vi "insert standard into cycle.vi"(1 "error out 2":errorcluster) -> (0 "error out":errorcluster)   [LabVIEW 2016]
panel:
  out "Array 2":dbl[][](array[numeric])
  out "Array":dbl[](array[numeric])
  out "sequence  Result":dbl[][](array[numeric])
  out "cycle results dbl":dbl[][](array[numeric])
  out "cycle results labels":string[](array[string])
  out "Cycle data by position":dbl[][][](array[numeric])
  out "Final Result":string[][](array[string])
  out "cycle result header":string[](array[string])
  out "sequence result header":string[](array[string])
  out "Final result header":string[](array[string])
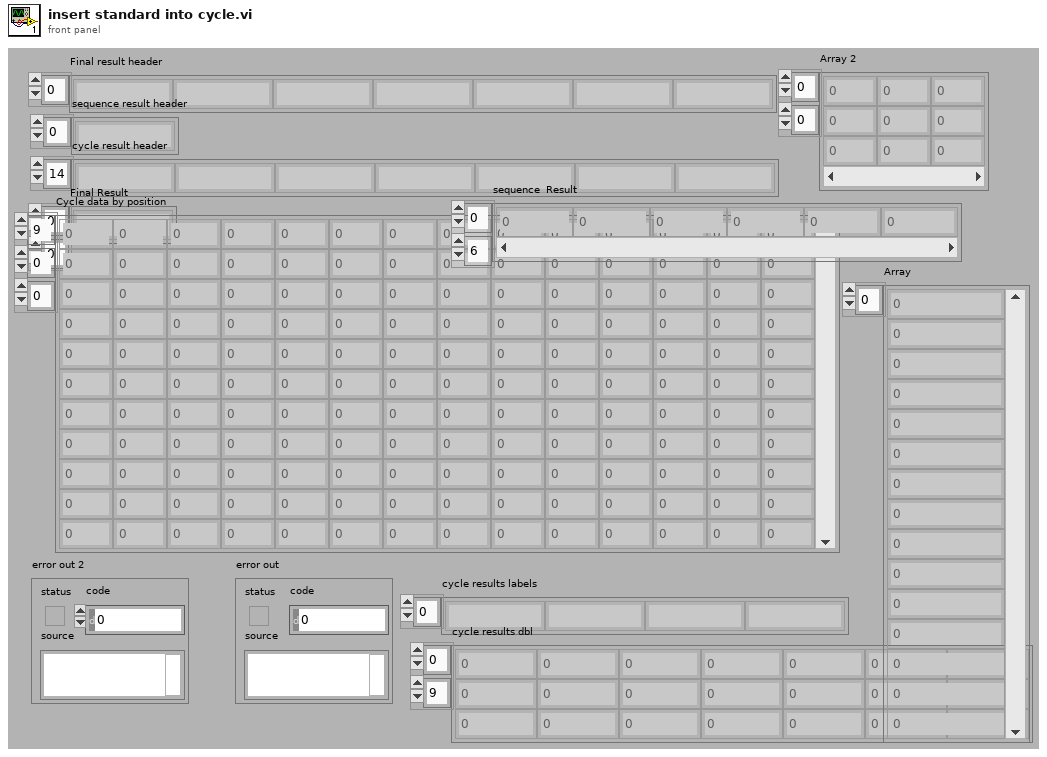
[diagram p1: front panel]
types:
  T1 = typedef "cycle results control.ctl" = cluster{"sample info":string[][], "cycle results labels":string[], "cycle results dbl":dbl[][]}
  T2 = typedef "data control cluster.ctl" = cluster{"Final result header":string[], "sequence result header":string[], "cycle result header ":string[], "Final Result":string[][], "sequence  Result":dbl[][], "Cycle data by seq":dbl[][][], "Cycle data by position":dbl[][][], "Final seq  Result":dbl[][], "only specific type":dbl[][]}
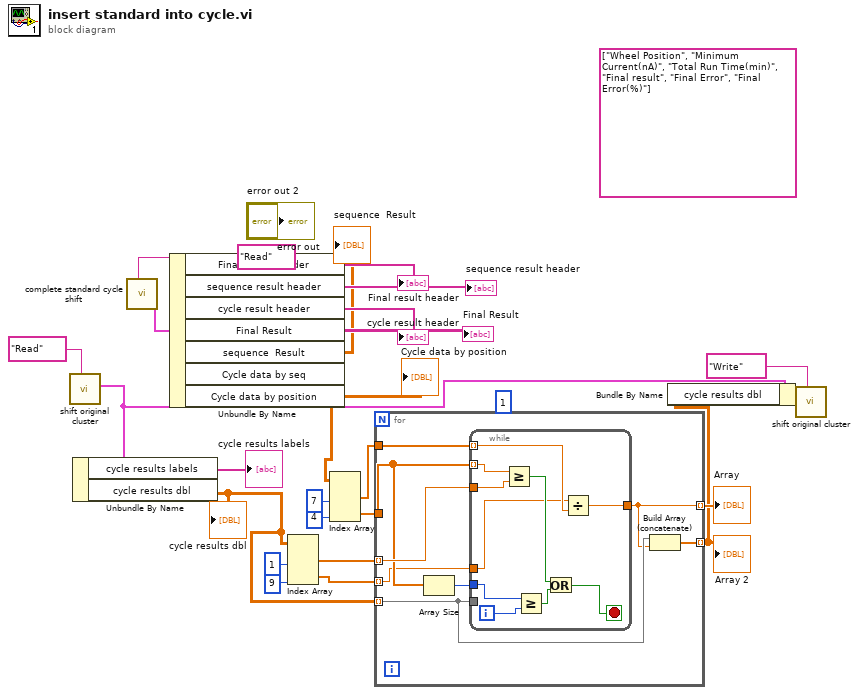
[diagram p0: block diagram]
diagram:
  (unwired) string[] ["Wheel Position", "Minimum Current(nA)", "Total Run Time(min)", "Final result", "Final Error", "Final Error(%)"]
  (unwired) 1 ("disabled index (col)")
  n1 = call "shift original cluster.vi"("read write shift"="Read") -> ("cycle results cluster out"=w3:T1)  [unwired: 9 in, 1 out]
  n2 = Unbundle By Name(w3) -> ("cycle results labels"=→"cycle results labels":string[], "cycle results dbl"=w10:dbl[][])
  "cycle results dbl" <- w10
  n3 = call "complete standard cycle shift.vi"("read write shift"="Read") -> ("DATA CLUSTER out"=w23:T2)  [unwired: 9 in, 1 out]
  n4 = Unbundle By Name(w23) -> ("Final result header"=→"Final result header":string[], "sequence result header"=→"sequence result header":string[], "cycle result header"=→"cycle result header":string[], "Final Result"=→"Final Result":string[][], "sequence  Result"=w14:dbl[][], "Cycle data by position"=→"Cycle data by position":dbl[][][])  [unwired: 1 out]
  "sequence  Result" <- w14
  n5 = Index Array(array=w10, index (col) #1=1 ("disabled index (col)"), index (col) #2=9 ("index (col)")) -> (element #1=w11:dbl[], element #2=w6:dbl[])  [unwired: 2 in]
  n6 = Index Array(array=w14, index (col) #1=7 ("disabled index (col)"), index (col) #2=4 ("index (col)")) -> (element #1=w9:dbl[], element #2=w8:dbl[])  [unwired: 2 in]
  n7 = for {
    tunnel: w11 -> [w33] mode=indexing
    tunnel: w10 -> [w28] mode=indexing
    tunnel: w9 -> [w32]
    tunnel: w8 -> [w30]
    tunnel: w6 -> [w29] mode=indexing
    tunnel: [w27] -> w5 mode=indexing
    tunnel: [w26] -> w2 mode=indexing
    n8 = Array Size(array=w30) -> (size(s)=w31:i32)
    n9 = while {
      tunnel: w33 -> [w40]
      tunnel: w32 -> [w36] mode=indexing
      tunnel: w30 -> [w41] mode=indexing
      tunnel: w28 -> [_]
      tunnel: w31 -> [w42]
      tunnel: w29 -> [w35]
      tunnel: [w34] -> w27
      i -> [w43]
      stop <- w37 stop-if-true
      n10 = Greater Or Equal?(x=w41, y=w40) -> (x >= y?=w38:bool)
      n11 = Greater Or Equal?(x=w42, y=w43) -> (x >= y?=w39:bool)
      n12 = Or(x=w38, y=w39) -> (x .or. y?=w37:bool)
      n13 = Divide(x=w35, y=w36) -> (x/y=w34:dbl)
    }
    n14 = Build Array (concatenate)(w28, w27) -> (w26:dbl[])
  }
  "Array" <- w5
  "Array 2" <- w2
  n15 = Bundle By Name(cluster=w3, "cycle results dbl"=w2) -> (w1:T1)
  n16 = call "shift original cluster.vi"("read write shift"="Write", "cycle results cluster In"=w1) -> ()  [unwired: 8 in, 2 out]
  "error out" <- "error out 2"
